vi "Write Global Stop.vi"(10 "Global Stop":T1, 11 "Template in":refnum<class "Template.lvclass">) -> (3 "Template out":refnum<class "Template.lvclass">)   [LabVIEW 2020, in "Template.lvlib" / "Template.lvclass"]
uses:
  Template.lvclass
  typedefs/global stop.ctl
  Template.lvclass/Template.ctl
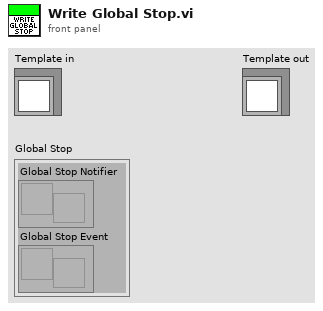
[diagram p1: front panel]
types:
  T1 = typedef "Template.lvlib/Template.lvclass/global stop.ctl" = cluster{"Global Stop Notifier":refnum<notifier>, "Global Stop Event":refnum<user-event>}
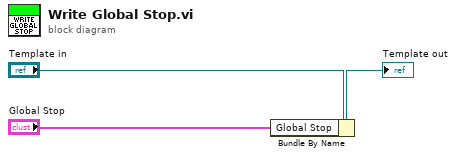
[diagram p0: block diagram]
diagram:
  n1 = Bundle By Name(cluster="Template in", "Global Stop"="Global Stop") -> (→"Template out":refnum<class "Template.lvclass">)
